vi "Postgresql Connect.vi"(5 "SqlMapper Type":refnum<class "SqlMapper.lvclass">, 8 "error in (no error)":errorcluster, 10 "Connection String":string) -> (0 "error out":errorcluster, 3 "SqlMapper out":refnum<class "SqlMapper.lvclass">)   [LabVIEW 2020, in "ORM_DBC_Npgsql.lvlib" / "DBC.lvclass"]
uses:
  DBC.lvclass
  <vilib>/Viviota/shared/ORM.lvlibp/ORM/SqlMapper/SqlMapper.lvclass
  C:/Program Files/National Instruments/LabVIEW 2024/vi.lib/Viviota/shared/ORM.lvlibp/ORM/DbConnection/DbConnection.lvclass
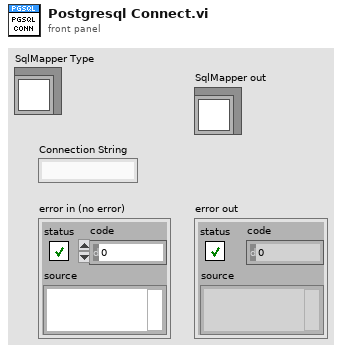
[diagram p1: front panel]
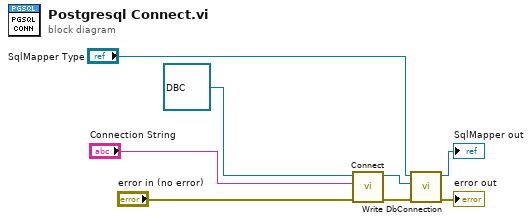
[diagram p0: block diagram]
diagram:
  n1 = call-dynamic "Connect.vi"("error in (no error)"="error in (no error)", "Connection String"="Connection String", "PostgresqlConnection in"=refnum<class "DBC.lvclass"> refnum ("PostgresqlConnection.lvclass")) -> ("error out"=w4:errorcluster, "PostgresqlConnection out"=w2:refnum<class "DBC.lvclass">)  [unwired: 7 in]
  n2 = call <vilib>:"Write DbConnection.vi"("error in (no error)"=w4, "Dapper.lvlib:DbConnection.lvclass"=w2, "SqlMapper in"="SqlMapper Type") -> ("error out"=→"error out":errorcluster, "SqlMapper out"=→"SqlMapper out":refnum<class "SqlMapper.lvclass">)  [unwired: 7 in]
